vi "test Read Message (TCP) Shares Timeout.vi"(8 "error in (no error)":errorcluster, 11 "TestCase in":refnum<class "TCP API Tests.lvclass">) -> (0 "error out":errorcluster, 3 "TestCase out":refnum<class "TCP API Tests.lvclass">)   [LabVIEW 2013, in "TCP API Tests.lvclass"]
uses:
  TCP API Tests.lvclass
  vi.lib/NI/STM/TCP/TCP Read Options.ctl
  vi.lib/NI/STM/TCP/TCP Data Info.ctl
  vi.lib/NI/STM/TCP/Write Meta Data (TCP Ref).vi
  vi.lib/NI/STM/TCP/Read Meta Data (TCP Ref).vi
  vi.lib/NI/STM/TCP/Write Meta Data (TCP Clst).vi
  vi.lib/NI/STM/TCP/Read Meta Data (TCP Clst).vi
  <vilib>/addons/_JKI Toolkits/VI Tester/TestCase.llb/TestCase.lvclass
  vi.lib/NI/STM/NI STM.lvlib
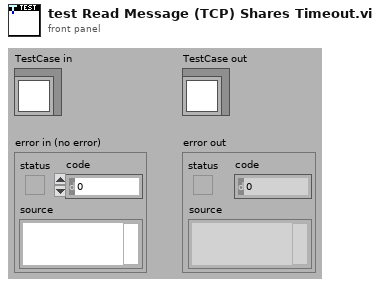
[diagram p1: front panel]
types:
  T1 = typedef "NI STM.lvlib/TCP Data Info.ctl" = cluster{"data size":i32, "retry read":bool}
  T2 = typedef "NI STM.lvlib/TCP Read Options.ctl" = cluster{"ignore timeout error":bool, "timeout ms (1000)":i32}
  T3 = typedef "NI STM.lvlib/TCP Connection Info.ctl" = cluster{"connection ID":refnum<k5>, "meta data":T4[]}
  T4 = typedef "NI STM.lvlib/MetaDataElement.ctl" = string
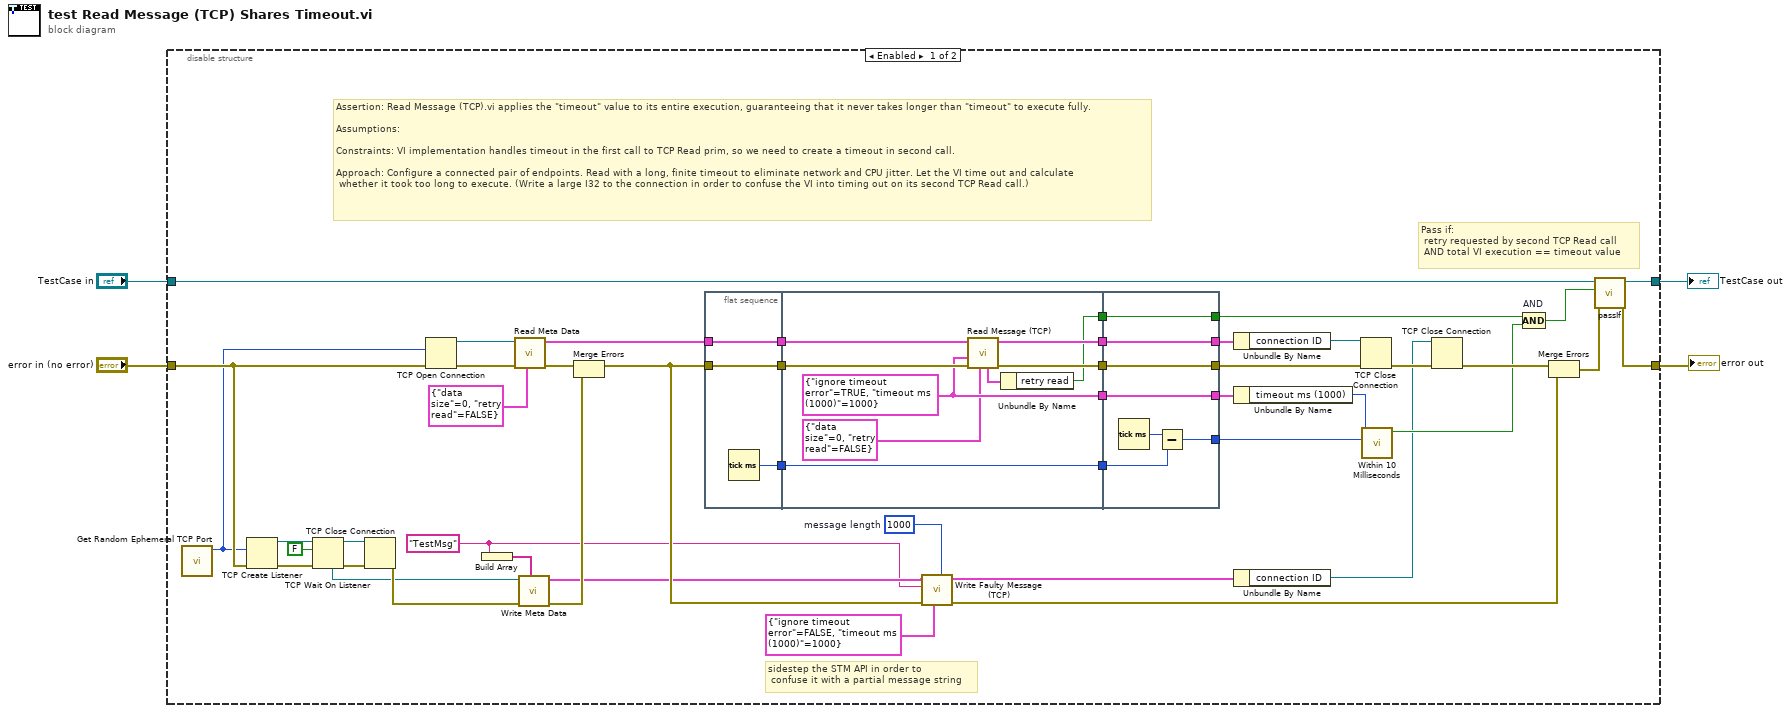
[diagram p0: block diagram]
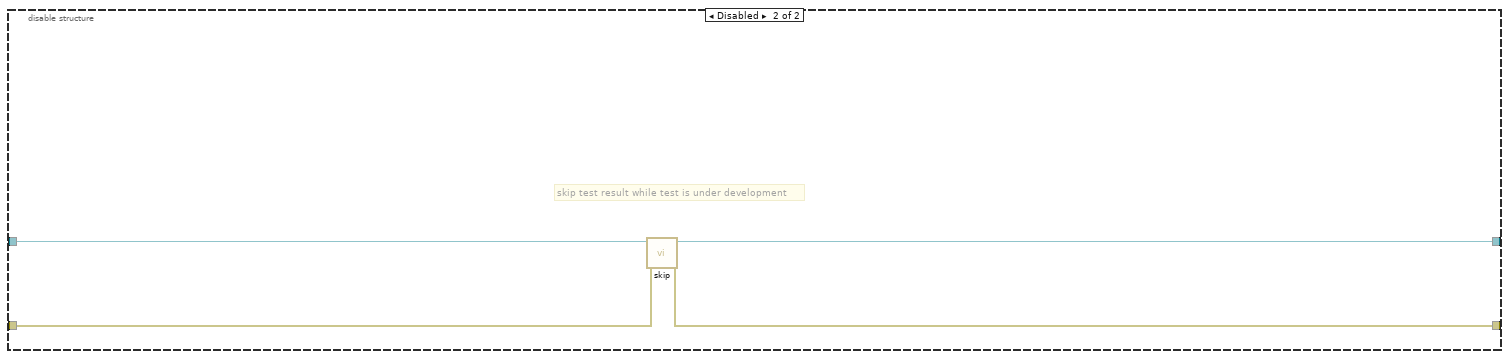
[diagram p2: hidden frame]
diagram:
  n1 = disable-structure shown="Enabled" {
    disable-tunnel: "TestCase in" -> [w51 w74]
    disable-tunnel: [w50 w72] -> w1
    disable-tunnel: [w49 w73] -> w3
    disable-tunnel: "error in (no error)" -> [w7 w71]
    frame Enabled {
      w15 = "TestMsg" ("Meta Element")
      w21 = i64 1000  # message length
      # "Pass if:\n retry requested by second TCP Read call\n AND total VI execution == timeout value"
      # "sidestep the STM API in order to\n confuse it with a partial message string"
      # "Assertion: Read Message (TCP).vi applies the \"timeout\" value to its entire execution, guaranteeing that it never takes longer than \"timeout\" to execute fully.\n\nAssumptions: \n\nConstraints: VI implementation handles timeout in the first call to TCP Read prim, so we need to create a timeout in second call.\n\nApproach: Configure a connected pair of endpoints. Read with a long, finite timeout to eliminate network and CPU jitter. Let the VI time out and calculate\n whether it took too long to execute. (Write a large I32 to the connection in order to confuse the VI into timing out on its second TCP Read call.)"
      n2 = call "Get Random Ephemeral TCP Port.vi"() -> ("ephemeral TCP port"=w6:u16)  [unwired: 11 in]
      n3 = TCP Create Listener(8:w7, 10:w6) -> (0:w12:errorcluster, 3:w11:refnum<k5>)  [unwired: 3 in, 1 out]
      n4 = TCP Wait On Listener(8:w12, 10:FALSE, 11:w11) -> (0:w13:errorcluster, 3:w10:refnum<k5>, 4:w5:refnum<k5>)  [unwired: 1 in, 2 out]
      n5 = TCP Close Connection(connection ID=w10, error in (no error)=w13) -> (error out=w8:errorcluster)  [unwired: 1 in, 1 out]
      n6 = TCP Open Connection(remote port or service name=w6, error in (no error)=w7) -> (connection ID=w48:refnum<k5>, error out=w32:errorcluster)  [unwired: 3 in]
      n7 = Build Array(w15) -> (w16:string[])
      n8 = call-poly "Read Meta Data.vi"("prev data info"=T1 {"data size"=0, "retry read"=FALSE}, "error in"=w32, "connection ID"=w48) -> ("error out"=w47:errorcluster, "connection info out"=w45:T3)  [unwired: 1 in, 6 out]
      n9 = call-poly "Write Meta Data.vi"("meta data"=w16, "error in"=w8, "connection ID"=w5) -> ("error out"=w31:errorcluster, "connection info out"=w19:T3)  [unwired: 2 in, 5 out]
      n10 = Merge Errors(w47, w31) -> (w22:errorcluster)
      n11 = flat-sequence {
        tunnel: w45 -> [w53]
        tunnel: w22 -> [w54]
        tunnel: [w54] -> w44
        tunnel: [w53] -> w43
        tunnel: [w52] -> w40
        tunnel: w44 -> [w63]
        tunnel: w43 -> [w62]
        tunnel: [w57] -> w42
        tunnel: [w61] -> w41
        tunnel: w40 -> [w61]
        tunnel: [w59] -> w39
        tunnel: [w60] -> w37
        tunnel: [w55] -> w29
        tunnel: [w70] -> w46
        tunnel: w42 -> [w70]
        tunnel: w41 -> [w68]
        tunnel: w39 -> [w67]
        tunnel: [w67] -> w38
        tunnel: [w66] -> w28
        tunnel: [w65] -> w36
        tunnel: w37 -> [w65]
        tunnel: [w64] -> w26
        tunnel: w29 -> [w64]
        frame #0 {
          n12 = Tick Count (ms)() -> (millisecond timer value=w52:u32)
        }
        frame #1 {
          w59 = T2 {"ignore timeout error"=TRUE, "timeout ms (1000)"=1000} ("options")
          n13 = call "Read Message (TCP).vi"("prev data info"=T1 {"data size"=0, "retry read"=FALSE}, "error in"=w63, "options"=w59, "connection info in"=w62) -> ("error out"=w57:errorcluster, "connection info out"=w60:T3, "data info"=w56:T1)  [unwired: 2 in, 3 out]
          n14 = Unbundle By Name(w56) -> ("retry read"=w55:bool)
        }
        frame #2 {
          n15 = Tick Count (ms)() -> (millisecond timer value=w69:u32)
          n16 = Subtract(x=w69, y=w68) -> (x-y=w66:u32)
        }
      }
      n17 = call "Write Faulty Message (TCP).vi"("message length [bytes] (-1: calculate)"=w21, "options"=T2 {"ignore timeout error"=FALSE, "timeout ms (1000)"=1000}, "error in"=w22, "name (\"\")"=w15, "connection info in"=w19) -> ("error out"=w23:errorcluster, "connection info out"=w18:T3)  [unwired: 5 in]
      n18 = Unbundle By Name(w36) -> ("connection ID"=w35:refnum<k5>)
      n19 = Unbundle By Name(w38) -> ("timeout ms (1000)"=w27:i32)
      n20 = Unbundle By Name(w18) -> ("connection ID"=w17:refnum<k5>)
      n21 = TCP Close Connection(connection ID=w35, error in (no error)=w46) -> (error out=w34:errorcluster)  [unwired: 1 in, 1 out]
      n22 = call "Within 10 Milliseconds.vi"("milliseconds 2"=w28, "milliseconds 1"=w27) -> ("within 10 ms"=w25:bool)  [unwired: 9 in]
      n23 = TCP Close Connection(connection ID=w17, error in (no error)=w34) -> (error out=w33:errorcluster)  [unwired: 1 in, 1 out]
      n24 = Compound Arithmetic op=AND "AND"(w26, w25) -> (w24:bool)
      n25 = Merge Errors(w33, w23) -> (w30:errorcluster)
      n26 = call-dynamic "passIf.vi"("error in (no error)"=w30, "pass"=w24, "TestCase in"=w51) -> ("error out"=w49:errorcluster, "TestCase out"=w50:refnum<class "TCP API Tests.lvclass">)  [unwired: 7 in]
    }
    frame Disabled {
      # "skip test result while test is under development"
      n27 = call <vilib>:"skip.vi"("error in (no error)"=w71, "TestCase in"=w74) -> ("error out"=w73:errorcluster, "TestCase out"=w72:refnum<class "TCP API Tests.lvclass">)  [unwired: 8 in]
    }
  }
  "error out" <- w3
  "TestCase out" <- w1
